vi "Check raw holography data.vi"(9 "Target SD (8-bit)":dbl=20.0, 10 "Every nth frame":i32=50, 11 "Input movie":path) -> ()   [LabVIEW 2018]
uses:
  <vilib>/Analysis/NI_AALBase.lvlib
panel:
  out "Write frame #":i32
  out "Number of frames in original movie":u32
  out "Read frame #":i32
  out "Median row":i32
  out "Frames in new stack":i32
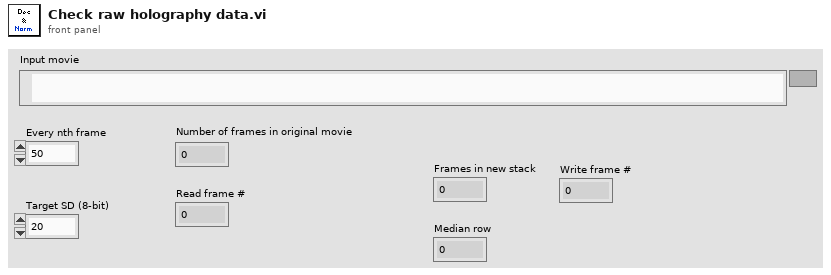
[diagram p1: front panel]
types:
  T1 = typedef "AviRefnum.ctl" = refnum<k1>
  T2 = cluster{"width":u32, "height":u32, "framesPerSecond":u32, "compressionFilter":string, "hasData":bool}
  T3 = typedef "IMAQ Image.ctl" = refnum<image>
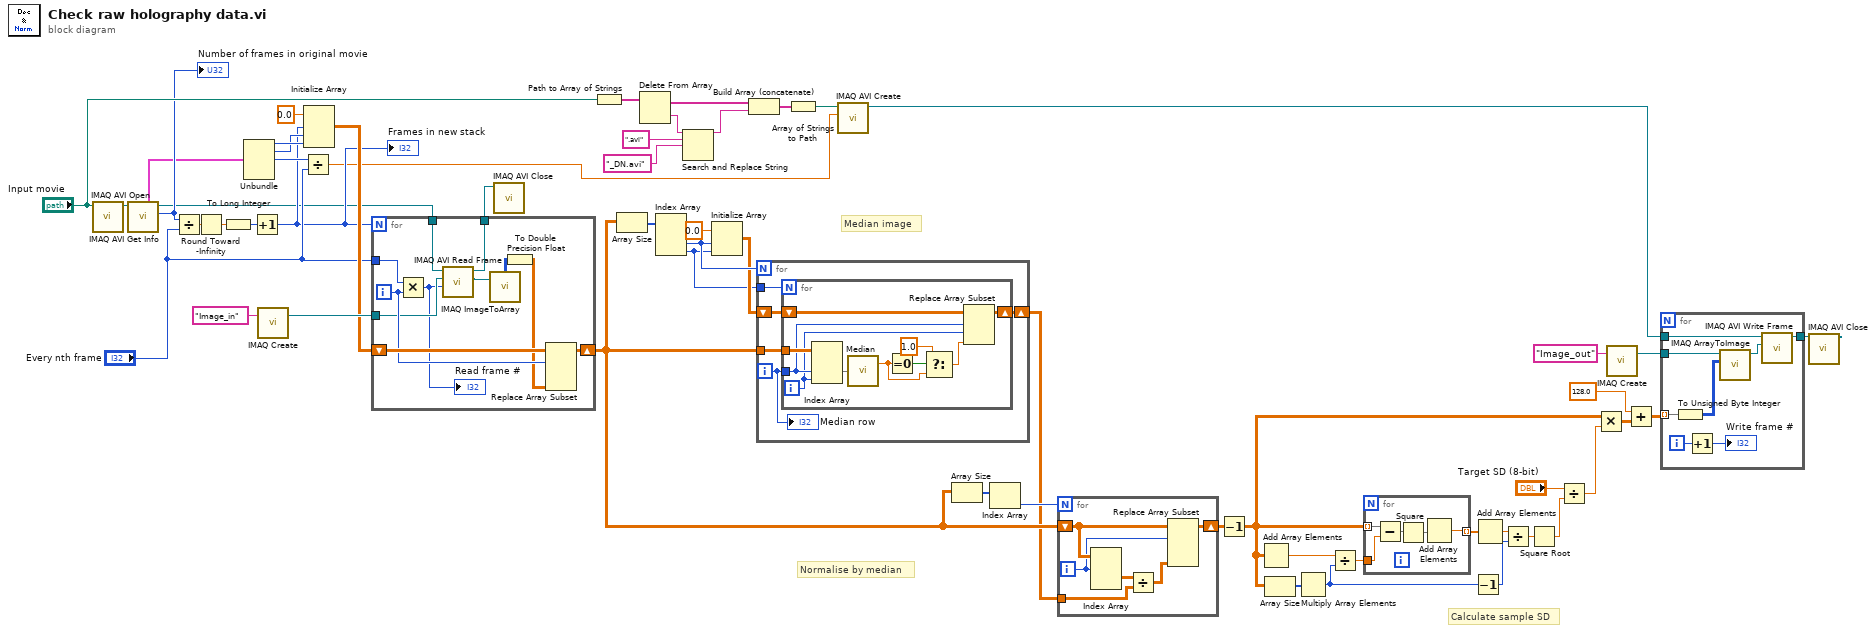
[diagram p0: block diagram]
diagram:
  # "Calculate sample SD"
  # "Normalise by median"
  # "Median image"
  n1 = call "IMAQ AVI Open"("AVI Path"="Input movie") -> ("Avi Refnum"=w11:T1)  [unwired: 9 in, 1 out]
  n2 = call "IMAQ AVI Get Info"("Avi Refnum"=w11) -> ("Number of Frames"=w9:u32, "Avi Refnum (duplicate)"=w7:T1, "Frame Data"=w8:T2)  [unwired: 6 in, 2 out]
  "Number of frames in original movie" <- w9
  n3 = Divide(x=w9, y="Every nth frame") -> (x/y=w56:dbl)
  n4 = Round Toward -Infinity(1:w56) -> (0:w15:dbl)
  n5 = To Long Integer(number=w15) -> (32bit integer=w14:i32)
  n6 = Unbundle(w8) -> ("width"=w53:u32, "height"=w52:u32, "framesPerSecond"=w20:u32)  [unwired: 2 out]
  n7 = Increment(x=w14) -> (x+1=w12:i32)
  "Frames in new stack" <- w12
  n8 = call "IMAQ Create"("Image Name"="Image_in") -> ("New Image"=w54:T3)  [unwired: 4 in, 1 out]
  n9 = Divide(x=w20, y="Every nth frame") -> (x/y=w5:dbl)
  n10 = Initialize Array(0.0 ("element"), w12, w52, w53) -> (w50:dbl[][][])
  n11 = for {
    N: w12 -> [_]
    tunnel: w7 -> [w61]
    tunnel: "Every nth frame" -> [w67]
    tunnel: w54 -> [w60]
    tunnel: [w58] -> w6
    shift-right: [w65] -> w45
    shift-left: w50 -> [w66]
    i -> [w64]
    n12 = Multiply(x=w67, y=w64) -> (x*y=w59:i32)
    "Read frame #" <- w59
    n13 = call "IMAQ AVI Read Frame"("Frame Number"=w59, "Image"=w60, "Avi Refnum"=w61) -> ("Image Out"=w57:T3, "Avi Refnum (duplicate)"=w58:T1)  [unwired: 5 in, 2 out]
    n14 = call "IMAQ ImageToArray"("Image"=w57) -> ("Image Pixels (U8)"=w62:u8[][])  [unwired: 3 in, 4 out]
    n15 = To Double Precision Float(number=w62) -> (double precision float=w63:dbl[][])
    n16 = Replace Array Subset(array=w66, new element=w63, index (dim 0)=w64) -> (w65:dbl[][][])  [unwired: 2 in]
  }
  n17 = call "IMAQ AVI Close"("Avi Refnum"=w6) -> ()  [unwired: 10 in, 1 out]
  n18 = Path to Array of Strings(0:"Input movie") -> (2:w27:string[])  [unwired: 1 out]
  n19 = Array Size(array=w45) -> (size(s)=w48:i32[])
  n20 = Delete From Array(array=w27) -> (deleted portion=w26:string, array with subset deleted=w23:string[])  [unwired: 2 in]
  n21 = Index Array(array=w48) -> (element #2=w47:i32, element #3=w13:i32)  [unwired: 3 in, 1 out]
  n22 = Search and Replace String(input string=w26, search string=".avi", replace string="_DN.avi" ("replace string (\"\")")) -> (result string=w22:string)  [unwired: 5 in, 3 out]
  n23 = Initialize Array(0.0 ("element"), w47, w13) -> (w46:dbl[][])
  n24 = Build Array (concatenate)(w23, w22) -> (w21:string[])
  n25 = for {
    N: w47 -> [_]
    tunnel: w45 -> [w69]
    tunnel: w13 -> [w72]
    shift-right: [w70] -> w1
    shift-left: w46 -> [w71]
    i -> [w68]
    n26 = for {
      N: w72 -> [_]
      shift-right: [w79] -> w70
      shift-left: w71 -> [w82]
      tunnel: w69 -> [w81]
      tunnel: w68 -> [w78]
      i -> [w77]
      n27 = Index Array(array=w81, index (dim 1)=w78, index (dim 2)=w77) -> (element=w80:dbl[])  [unwired: 1 in]
      n28 = call <vilib>:"Median.vi"("X"=w80) -> ("median"=w74:dbl)  [unwired: 1 out]
      n29 = Equal To 0?(x=w74) -> (x = 0?=w76:bool)
      n30 = Select(t=1.0, s=w76, f=w74) -> (s? t:f=w75:dbl)
      n31 = Replace Array Subset(array=w82, new element=w75, index (row)=w78, index (col)=w77) -> (w79:dbl[][])
    }
    "Median row" <- w68
  }
  n32 = Array of Strings to Path(0:w21) -> (2:w4:path)  [unwired: 1 in]
  n33 = call "IMAQ AVI Create"("Frames Per Second"=w5, "AVI Path"=w4) -> ("Avi Refnum"=w3:T1)  [unwired: 8 in, 1 out]
  n34 = Array Size(array=w45) -> (size(s)=w44:i32[])
  n35 = Index Array(array=w44) -> (element=w43:i32)  [unwired: 1 in]
  n36 = for {
    N: w43 -> [_]
    tunnel: w1 -> [w87]
    shift-right: [w85] -> w42
    shift-left: w45 -> [w86]
    i -> [w84]
    n37 = Index Array(array=w86, index (dim 0)=w84) -> (element=w88:dbl[][])  [unwired: 2 in]
    n38 = Divide(x=w88, y=w87) -> (x/y=w83:dbl[][])
    n39 = Replace Array Subset(array=w86, new element=w83, index (dim 0)=w84) -> (w85:dbl[][][])  [unwired: 2 in]
  }
  n40 = Decrement(x=w42) -> (x-1=w30:dbl[][][])
  n41 = Add Array Elements(numeric array=w30) -> (sum=w40:dbl)
  n42 = Array Size(array=w30) -> (size(s)=w41:i32[])
  n43 = Multiply Array Elements(1:w41) -> (0:w37:i32)
  n44 = Divide(x=w40, y=w37) -> (x/y=w39:dbl)
  n45 = for {
    tunnel: w30 -> [w92] mode=indexing
    tunnel: w39 -> [w93]
    tunnel: [w89] -> w38 mode=indexing
    n46 = Subtract(x=w92, y=w93) -> (x-y=w91:dbl[][])
    n47 = Square(x=w91) -> (x^2=w90:dbl[][])
    n48 = Add Array Elements(numeric array=w90) -> (sum=w89:dbl)
  }
  n49 = Decrement(x=w37) -> (x-1=w35:i32)
  n50 = Add Array Elements(numeric array=w38) -> (sum=w36:dbl)
  n51 = Divide(x=w36, y=w35) -> (x/y=w34:dbl)
  n52 = Square Root(x=w34) -> (sqrt(x)=w32:dbl)
  n53 = Divide(x="Target SD (8-bit)", y=w32) -> (x/y=w31:dbl)
  n54 = Multiply(x=w30, y=w31) -> (x*y=w29:dbl[][][])
  n55 = call "IMAQ Create"("Image Name"="Image_out") -> ("New Image"=w16:T3)  [unwired: 4 in, 1 out]
  n56 = Add(x=128.0 ("x/y"), y=w29) -> (x+y=w18:dbl[][][])
  n57 = for {
    tunnel: w18 -> [w101] mode=indexing
    tunnel: w3 -> [w97]
    tunnel: w16 -> [w100]
    tunnel: [w95] -> w2
    i -> [w98]
    n58 = To Unsigned Byte Integer(number=w101) -> (unsigned 8bit integer=w99:u8[][])
    n59 = Increment(x=w98) -> (x+1=→"Write frame #":i32)
    n60 = call "IMAQ ArrayToImage"("Image Pixels (U8)"=w99, "Image"=w100) -> ("Image Out"=w96:T3)  [unwired: 8 in, 1 out]
    n61 = call "IMAQ AVI Write Frame"("Image"=w96, "Avi Refnum"=w97) -> ("Avi Refnum (duplicate)"=w95:T1)  [unwired: 8 in, 1 out]
  }
  n62 = call "IMAQ AVI Close"("Avi Refnum"=w2) -> ()  [unwired: 10 in, 1 out]
